vi "Aspect Ratio Score 2016.vi"(10 "Aspect Fudge Factor":dbl=1.0, 11 "Rectangle Array ltrb":dbl[](array[numeric])=[2.22, 1.4]) -> (3 "Aspect Ratio Score":dbl)   [LabVIEW 2016]
doc: "Compare the ratio of the bounding box to that of the expected target. Score is in percent.\nFudge factor compensates for the cameras and camera modes that don't produce square pixels.\n\nSince inputs are particle measurements, the diagram doesn't expect to receive zero or negative values for either input."
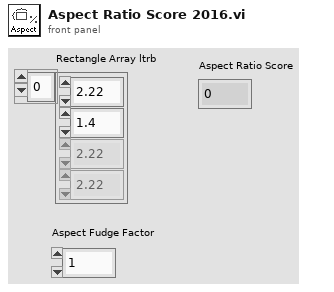
[diagram p1: front panel]
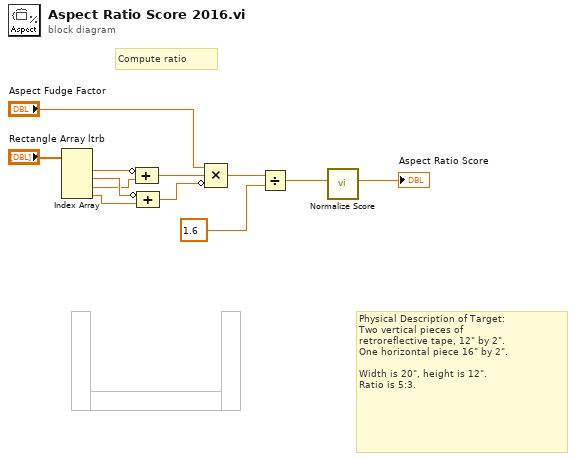
[diagram p0: block diagram]
diagram:
  # "Physical Description of Target:\nTwo vertical pieces of\nretroreflective tape, 12\" by 2\".\nOne horizontal piece 16\" by 2\".\n\nWidth is 20\", height is 12\".\nRatio is 5:3."
  # "Compute ratio"
  n1 = Index Array(array="Rectangle Array ltrb") -> (element #1=w8:dbl, element #2=w11:dbl, element #3=w9:dbl, element #4=w10:dbl)  [unwired: 4 in]
  n2 = Compound Arithmetic op=ADD(invert w8, w9) -> (w7:dbl)
  n3 = Compound Arithmetic op=ADD(invert w11, w10) -> (w6:dbl)
  n4 = Compound Arithmetic op=MULTIPLY("Aspect Fudge Factor", w7, invert w6) -> (w12:dbl)
  n5 = Divide(x=w12, y=1.6) -> (x/y=w2:dbl)
  n6 = call "Normalize Score.vi"("Value"=w2) -> ("Score"=→"Aspect Ratio Score":dbl)  [unwired: 10 in]
